vi "Calculate Sensor Angle.vi"(0 "DATA[4-5]":u8[](array[numeric]) format="%.0x") -> (14 "Degree0":dbl, 15 "Degree0 2":dbl)   [LabVIEW 2025]
panel:
  out "raw value 2":u16 format="%.0x"
  out "raw value":u16 format="%.0x"
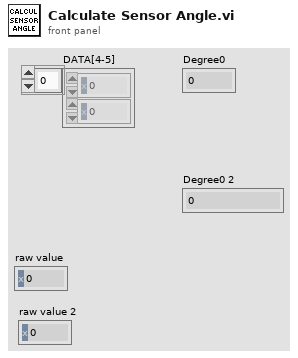
[diagram p1: front panel]
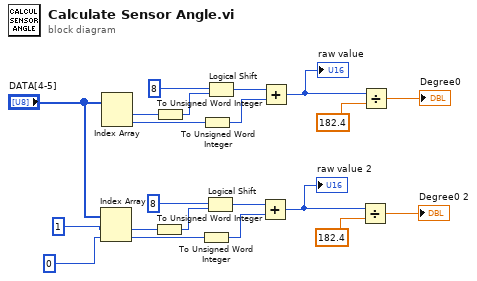
[diagram p0: block diagram]
diagram:
  n1 = Index Array(array="DATA[4-5]", index #1=1 ("index"), index #2=0 ("index")) -> (element #1=w7:u8, element #2=w5:u8)
  n2 = Index Array(array="DATA[4-5]") -> (element #1=w18:u8, element #2=w20:u8)  [unwired: 2 in]
  n3 = To Unsigned Word Integer(number=w7) -> (unsigned 16bit integer=w8:u16)
  n4 = To Unsigned Word Integer(number=w18) -> (unsigned 16bit integer=w17:u16)
  n5 = To Unsigned Word Integer(number=w5) -> (unsigned 16bit integer=w6:u16)
  n6 = To Unsigned Word Integer(number=w20) -> (unsigned 16bit integer=w19:u16)
  n7 = Logical Shift(y=u8 8 ("x"), x=w8) -> (x << y=w9:u16)
  n8 = Logical Shift(y=u8 8 ("x"), x=w17) -> (x << y=w16:u16)
  n9 = Add(x=w9, y=w6) -> (x+y=w10:u16)
  "raw value 2" <- w10
  n10 = Add(x=w16, y=w19) -> (x+y=w15:u16)
  "raw value" <- w15
  n11 = Divide(x=w10, y=182.4) -> (x/y=→"Degree0 2":dbl)
  n12 = Divide(x=w15, y=182.4) -> (x/y=→"Degree0":dbl)
